vi "Establish Serial Coms_v2.vi"(8 "error in (no error)":errorcluster, 11 "ControlBoard VISA":refnum<visa-resource-name>="ControlBoard") -> (0 "error out":errorcluster, 3 "ControlBoard VISA Out":refnum<visa-resource-name>)   [LabVIEW 2022 SP3]
doc: "This VI will loop until the Control Board VISA session is properly initialized. Ensure the name of the session matches the name of the Control Board VISA Com in NI MAX"
uses:
  <vilib>/Instr/_visa.llb/VISA Configure Serial Port (Instr).vi
panel:
  out "Loop Error?":errorcluster
  in  "stop":bool
  out "Instructional Message":string
  out "Unsuccesful Attempts to connect":i32
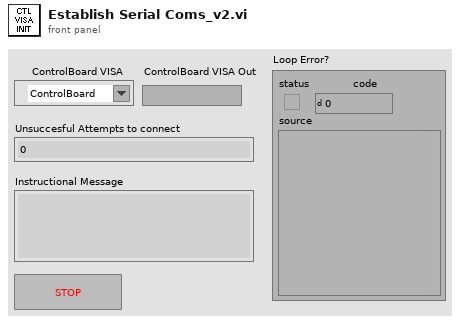
[diagram p1: front panel]
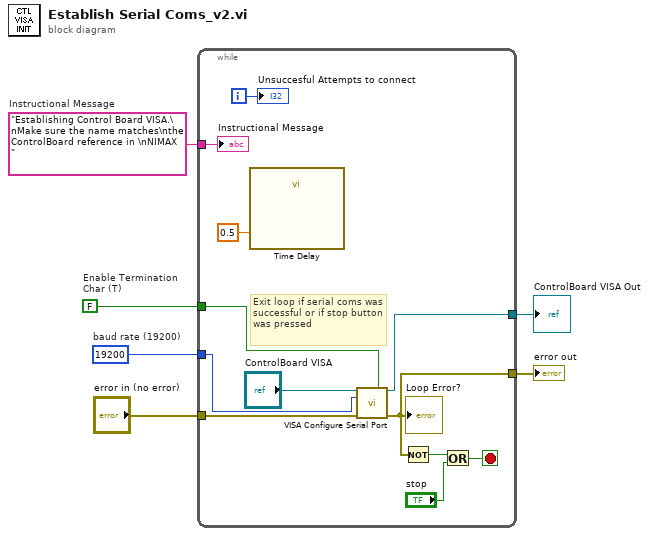
[diagram p0: block diagram]
diagram:
  w3 = "Establishing Control Board VISA.\nMake sure the name matches\nthe ControlBoard reference in \nNIMAX  "  # Instructional Message
  w4 = FALSE  # Enable Termination Char (T)
  w5 = u32 19200  # baud rate (19200)
  n1 = while {
    tunnel: "error in (no error)" -> [w15]
    tunnel: w5 -> [w14]
    tunnel: w4 -> [w13]
    tunnel: w3 -> [w12]
    tunnel: [w10] -> w2
    tunnel: [w7] -> w1
    i -> [w17]
    stop <- w16 stop-if-true
    # "Exit loop if serial coms was successful or if stop button was pressed"
    n2 = call "Time Delay"("Delay Time (s)"=0.5) -> ()  [unwired: 10 in, 1 out]
    n3 = call-poly "VISA Configure Serial Port"("VISA resource name"="ControlBoard VISA", "Enable Termination\nChar (T)"=w13, "baud rate (9600)"=w14, "error in (no error)"=w15) -> ("VISA resource name out"=w10:refnum<visa-resource-name>, "error out"=w7:errorcluster)  [unwired: 10 in]
    "Loop Error?" <- w7
    n4 = Not(x=w7) -> (.not. x?=w18:bool)
    n5 = Or(x=w18, y="stop") -> (x .or. y?=w16:bool)
    "Unsuccesful Attempts to connect" <- w17
    "Instructional Message" <- w12
  }
  "error out" <- w1
  "ControlBoard VISA Out" <- w2
